vi "Ins34401Read_ver1.0.vi"(0 "VISA session":refnum<visa-resource-name>, 1 "error out":errorcluster) -> (2 "VISA session 2":refnum<visa-resource-name>, 3 "Numeric":dbl, 4 "error out 2":errorcluster)   [LabVIEW 2012]
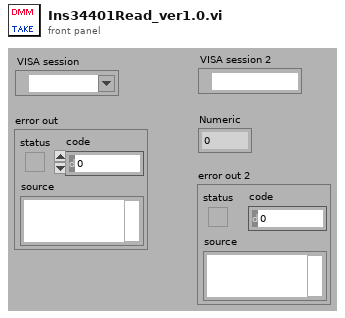
[diagram p1: front panel]
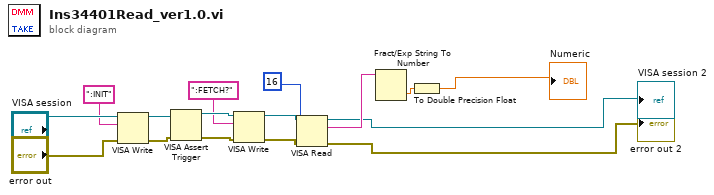
[diagram p0: block diagram]
diagram:
  n1 = VISA Write(VISA resource name="VISA session", write buffer=":INIT", error in (no error)="error out") -> (VISA resource name out=w9:refnum<visa-resource-name>, error out=w10:errorcluster)  [unwired: 1 out]
  n2 = VISA Assert Trigger(8:w10, 11:w9) -> (0:w3:errorcluster, 3:w4:refnum<visa-resource-name>)  [unwired: 1 in]
  n3 = VISA Write(VISA resource name=w4, write buffer=":FETCH?", error in (no error)=w3) -> (VISA resource name out=w13:refnum<visa-resource-name>, error out=w14:errorcluster)  [unwired: 1 out]
  n4 = VISA Read(VISA resource name=w13, byte count=u32 16, error in (no error)=w14) -> (VISA resource name out=→"VISA session 2":refnum<visa-resource-name>, read buffer=w16:string, error out=→"error out 2":errorcluster)  [unwired: 1 out]
  n5 = Fract/Exp String To Number(string=w16) -> (number=w15:dbl)  [unwired: 3 in, 1 out]
  n6 = To Double Precision Float(number=w15) -> (double precision float=→"Numeric":dbl)
